vi "temp_seq_09_4.vi"(0 "master":i32, 1 "shutdown":i32, 3 "Tr_orTj":i32, 5 "pause":i32, 7 "adjust":dbl, 9 "TempParams":dbl[](array[numeric])=[20.0, 35.0, 45.0, 20.0, 20.0, 35.0, 45.0, 20.0, 20.0, 20.0, 20.0, 20.0, 20.0, 20.0, 20.0, 40.0, 2.0, 1.0], 11 "TimeParams":i32[](array[numeric])=[1, 1, 1, 1, 1], 12 "port":i32=9, 13 "reset":i32, 14 "manual":i32) -> (4 "Tr":dbl, 6 "start_time":dbl, 10 "params":dbl[](array[numeric]), 15 "Waveform Chart":dynamicdata(graph))   [LabVIEW 2015]
uses:
  BERTTA.dll
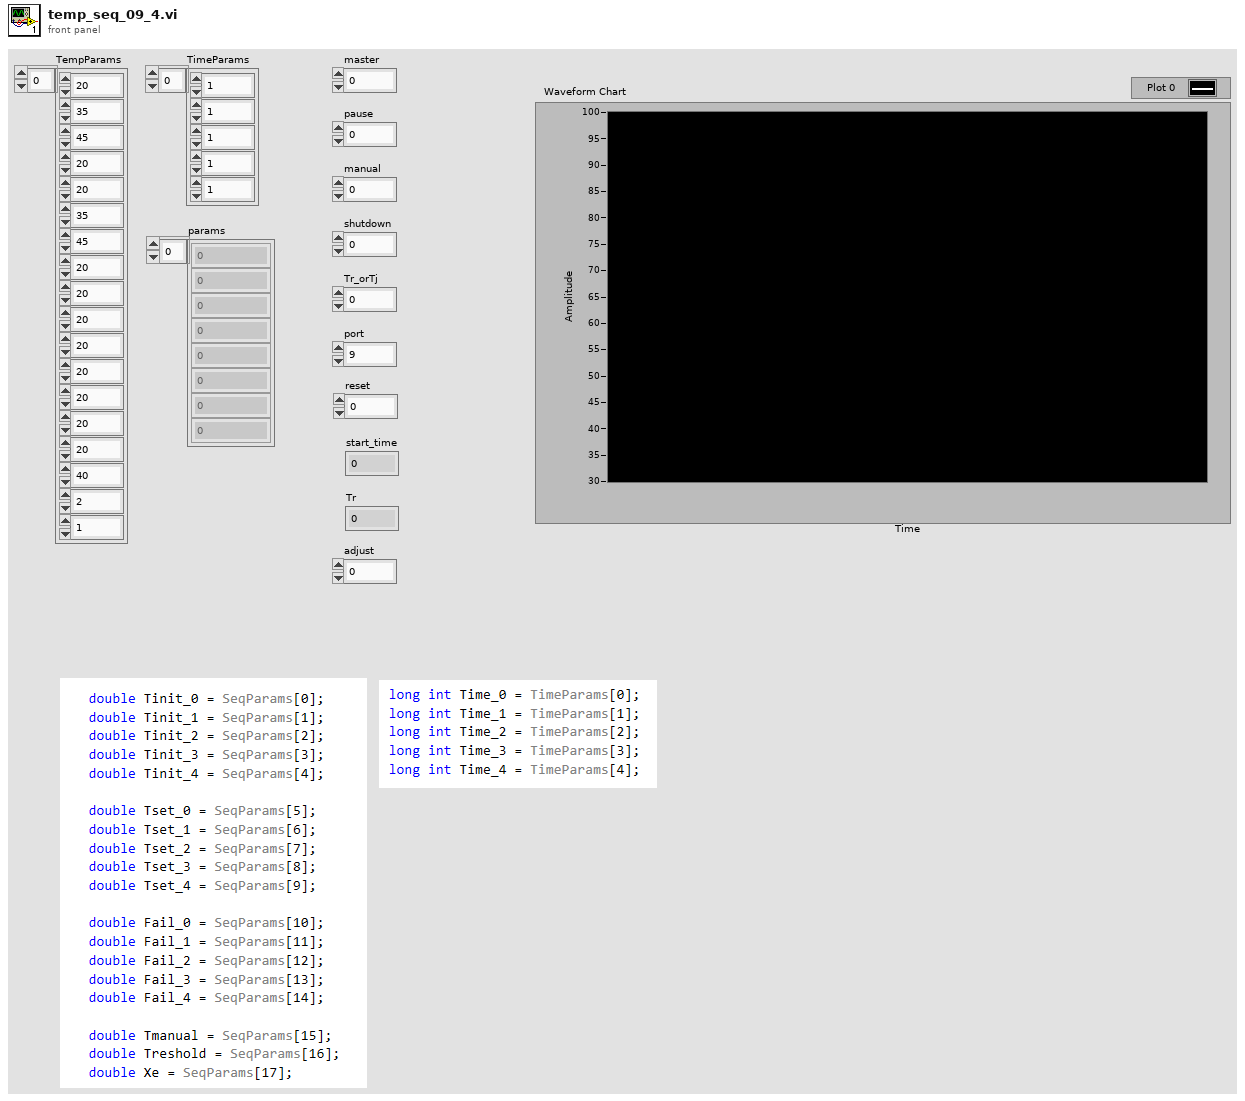
[diagram p1: front panel]
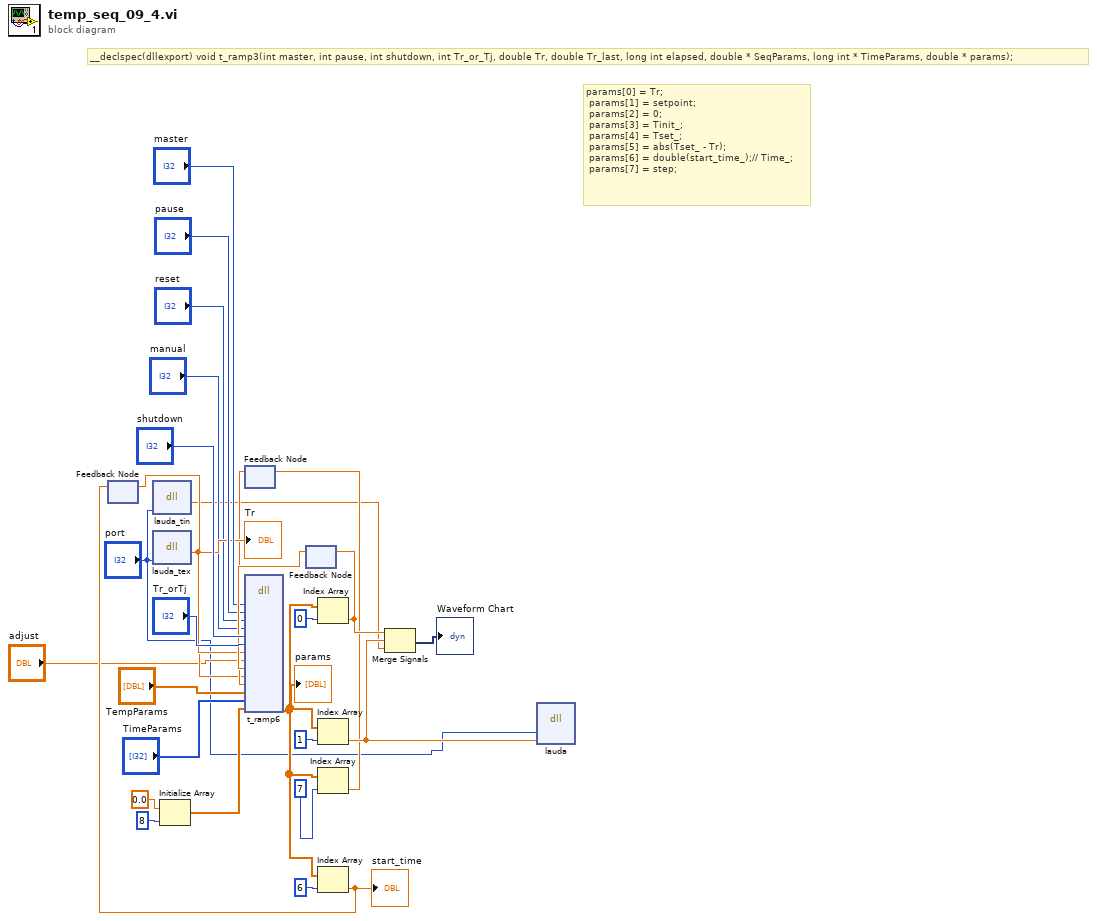
[diagram p0: block diagram]
diagram:
  # "params[0] = Tr;\n\tparams[1] = setpoint;\n\tparams[2] = 0;\n\tparams[3] = Tinit_;\n\tparams[4] = Tset_;\n\tparams[5] = abs(Tset_ - Tr);\n\tparams[6] = double(start_time_);// Time_;\n\tparams[7] = step;"
  # "__declspec(dllexport) void t_ramp3(int master, int pause, int shutdown, int Tr_or_Tj, double Tr, double Tr_last, long int elapsed, double * SeqParams, long int * TimeParams, double * params);"
  n1 = feedback #1() -> (w6:dbl)  [unwired: 1 in]
  n2 = dll-call lib="C:/Users/shresplab/OneDrive - Kemira Oyj/Documents/Visual Studio 2017/Projects/Bertta/BERTTA/x64/Debug/BERTTA.dll" fn="lauda_tin"("port"="port") -> ("return type"=w1:dbl)  [unwired: 4 in, 2 out]
  n3 = dll-call lib="C:/Users/shresplab/OneDrive - Kemira Oyj/Documents/Visual Studio 2017/Projects/Bertta/BERTTA/x64/Debug/BERTTA.dll" fn="lauda_tex"("port"="port") -> ("return type"=w16:dbl)  [unwired: 4 in, 2 out]
  "Tr" <- w16
  n4 = Initialize Array(0.0 ("element"), 8 ("dimension size")) -> (w22:dbl[])
  n5 = feedback #2() -> (w10:dbl)  [unwired: 1 in]
  n6 = feedback #3() -> (w20:dbl)  [unwired: 1 in]
  n7 = dll-call lib="C:/Users/shresplab/OneDrive - Kemira Oyj/Documents/Visual Studio 2017/Projects/Bertta/BERTTA/x64/Debug/BERTTA.dll" fn="t_ramp6"("master"="master", "pause"="pause", "reset"="reset", "manual"="manual", "shutdown"="shutdown", "Tr_orTj"="Tr_orTj", "Tr"=w16, "adjust"="adjust", "Tr_last"=w20, "start_time"=w6, "step_previous"=w10, "SeqParams"="TempParams", "TimeParams"="TimeParams", "params"=w22) -> ("params"=w8:dbl[])  [unwired: 17 in, 2 out]
  "params" <- w8
  n8 = Index Array(array=w8, index=0) -> (element=w15:dbl)
  n9 = feedback-in #3(w15) -> ()
  n10 = Index Array(array=w8, index=1) -> (element=w14:dbl)
  n11 = Index Array(array=w8, index=7) -> (element=w11:dbl)
  n12 = feedback-in #2(w11) -> ()
  n13 = Index Array(array=w8, index=6) -> (element=w7:dbl)
  "start_time" <- w7
  n14 = feedback-in #1(w7) -> ()
  n15 = Merge Signals(w15, w14, w1) -> (→"Waveform Chart":dynamicdata)
  n16 = dll-call lib="C:/Users/shresplab/OneDrive - Kemira Oyj/Documents/Visual Studio 2017/Projects/Bertta/BERTTA/x64/Debug/BERTTA.dll" fn="lauda"("port"="port", "set_temp"=w14) -> ()  [unwired: 6 in, 2 out]
